vi "IO_Initialize.vi"(8 "error in (no error)":errorcluster, 9 "VISA resource name":refnum<visa-resource-name>, 11 "IT6932A in":refnum<class "IT6932A.lvclass">) -> (0 "error out":errorcluster, 3 "IT6932A out":refnum<class "IT6932A.lvclass">)   [LabVIEW 2023, in "IT6932A.lvclass"]
uses:
  IT6932A.lvclass
  IT6932A.lvclass/IT6932A.ctl
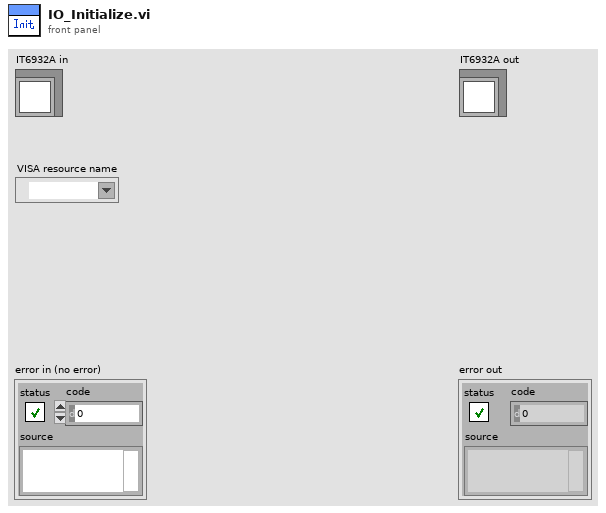
[diagram p1: front panel]
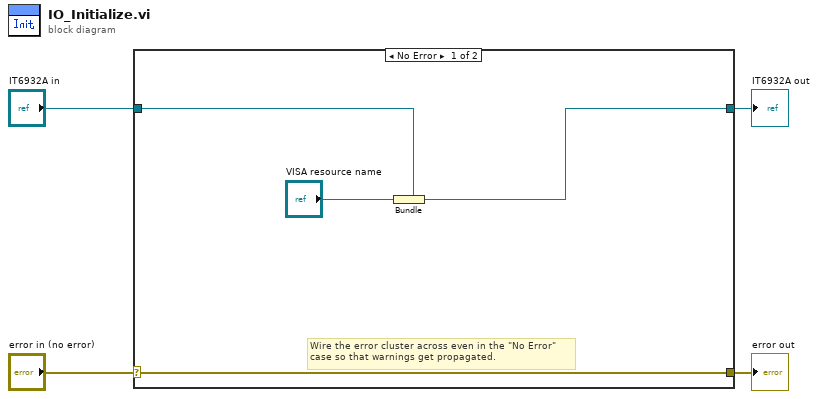
[diagram p0: block diagram]
diagram:
  n1 = case shown="No Error" "error in (no error)" {
    selector: "error in (no error)" -> [w8 w10]
    tunnel: [w8 w10] -> w3
    tunnel: [w6 w9] -> w1
    tunnel: "IT6932A in" -> [w7 w9]
    frame No Error {
      # "Wire the error cluster across even in the \"No Error\"\ncase so that warnings get propagated."
      n2 = Bundle(cluster=w7, "VISA resource name") -> (w6:refnum<class "IT6932A.lvclass">)
    }
    frame Error {
    }
  }
  "error out" <- w3
  "IT6932A out" <- w1
